vi "Auto Set Shooter.vi"(9 "Shot Type":dbl, 10 "Mode":dbl, 11 "Command":dbl) -> (3 "Finished?":bool)   [LabVIEW 2015]
uses:
  Common Code/Shooter Commands.ctl
  Common Code/Shoot Modes Enum.ctl
  Common Code/Shot Type.ctl
  Common Code/Drivetrain Modes.ctl
  Common Code/Change Detect Boolean.vi
  Robot Global Data.vi
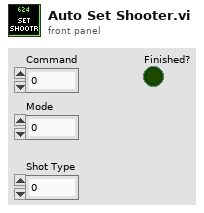
[diagram p1: front panel]
types:
  T1 = typedef "Drivetrain Commands.ctl" = cluster{"Y Power":dbl, "Turn Power":dbl, "2nd Gear?":bool, "Modes":T2, "Heading Target":dbl, "X Max Speed":dbl, "Y Max Speed":dbl, "X Min Speed":dbl, "Y Min Speed":dbl, "Y Target":dbl, "Max Accel":dbl, "Max Velocity":dbl, "Y Power 2":dbl, "Pivot Speed":dbl}
  T2 = typedef "Drivetrain Modes.ctl" = enum16{"Tank", "Climb", "Manual", "Goal Vision Targeting", "PID Distance Drive", "Hybrid", "Gyro Steer"}
  T3 = typedef "Shoot Modes Enum.ctl" = enum16{"Manual", "Safe", "Auto"}
  T4 = typedef "Shooter State Cluster.ctl" = cluster{"State":T5, "Left RPM":dbl, "Right RPM":dbl, "Shooter Ready?":bool, "Ball Loaded?":bool, "Current Angle":dbl, "Angle Motor Output":dbl, "Trigger Output":dbl, "Angle Ready?":bool, "RPM Ready?":bool, "Vision Ready?":bool, "Ball Loaded?":bool, "Mode":T3, "Shot Type":T6, "Pot Height":dbl, "Current Tripped Forward?":bool, "Current Tripped Backward?":bool, "Right Servo":i32, "Left Servo":i32, "IR Override":bool, "Intake Danger?":bool, "Intake Angle Ready?":bool}
  T5 = typedef "Shooter State.ctl" = enum16{"Idle", "Settle Ball", "Warmup", "Shooter Ready", "Shoot"}
  T6 = typedef "Shot Type.ctl" = enum16{"Batter Shot", "Corner Shot", "Cleat Shot", "Vision Shot", "Deep Middle Shot"}
  T7 = typedef "Shooter Commands.ctl" = enum16{"Idle", "Prime Shooter", "Shoot"}
  T8 = typedef "Shooter Command Cluster.ctl" = cluster{"Command":T7, "Mode":T3, "Shot Type":T6, "Override Trigger Sensor":bool, "Override Angle?":bool, "Hide From Death":bool}
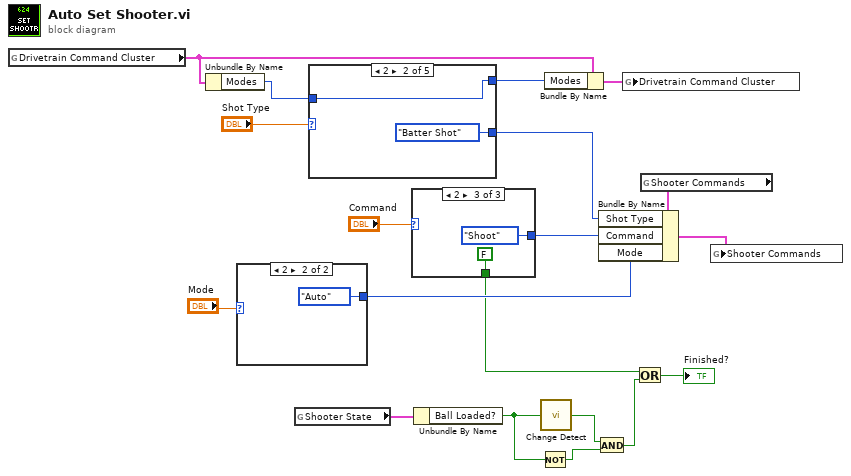
[diagram p0: block diagram]
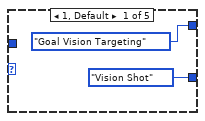
[diagram p2: hidden frame]
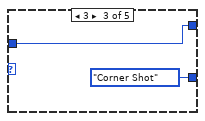
[diagram p3: hidden frame]
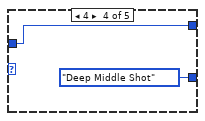
[diagram p4: hidden frame]
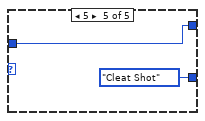
[diagram p5: hidden frame]
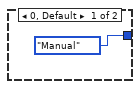
[diagram p6: hidden frame]
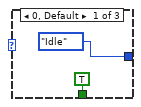
[diagram p7: hidden frame]
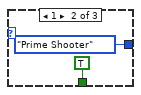
[diagram p8: hidden frame]
diagram:
  n1 = global read "Robot Global Data.vi" "Drivetrain Command Cluster"() -> (w16:T1)
  n2 = Unbundle By Name(w16) -> ("Modes"=w9:T2)
  n3 = case shown="2" "Mode" {
    tunnel: [Shoot_Modes_Enum."Manual" ("Mode") Shoot_Modes_Enum."Auto" ("Mode")] -> w12
    frame 0, Default {
    }
    frame 2 {
    }
  }
  n4 = global read "Robot Global Data.vi" "Shooter State"() -> (w7:T4)
  n5 = case shown="2" "Shot Type" {
    tunnel: [Shot_Type."Vision Shot" ("Shot Type") Shot_Type."Batter Shot" ("Shot Type") Shot_Type."Corner Shot" ("Shot Type") Shot_Type."Deep Middle Shot" ("Shot Type") Shot_Type."Cleat Shot" ("Shot Type")] -> w10
    tunnel: w9 -> [_ w25 w27 w28 w31]
    tunnel: [Drivetrain_Modes."Goal Vision Targeting" ("Modes") w25 w27 w28 w31] -> w8
    frame 1, Default {
    }
    frame 2 {
    }
    frame 3 {
    }
    frame 4 {
    }
    frame 5 {
    }
  }
  n6 = case shown="2" "Command" {
    tunnel: [Shooter_Commands."Idle" ("Command") Shooter_Commands."Prime Shooter" ("Command") Shooter_Commands."Shoot" ("Command")] -> w14
    tunnel: [TRUE TRUE FALSE] -> w1
    frame 0, Default {
    }
    frame 1 {
    }
    frame 2 {
    }
  }
  n7 = Unbundle By Name(w7) -> ("Ball Loaded?"=w6:bool)
  n8 = Not(x=w6) -> (.not. x?=w5:bool)
  n9 = call-poly "Change Detect.vi"("In"=w6) -> ("Changed?"=w4:bool)
  n10 = Bundle By Name(cluster=w16, "Modes"=w8) -> (w17:T1)
  n11 = And(x=w4, y=w5) -> (x .and. y?=w2:bool)
  n12 = global write "Robot Global Data.vi" "Drivetrain Command Cluster"(w17) -> ()
  n13 = Or(x=w1, y=w2) -> (x .or. y?=→"Finished?":bool)
  n14 = global read "Robot Global Data.vi" "Shooter Commands"() -> (w19:T8)
  n15 = Bundle By Name(cluster=w19, "Shot Type"=w10, "Command"=w14, "Mode"=w12) -> (w18:T8)
  n16 = global write "Robot Global Data.vi" "Shooter Commands"(w18) -> ()
